vi "create data folder.vi"(7 "Book name":string="book526", 8 "error in":errorcluster, 11 "Contour plot folder":path=path "C:/Users/gyue/Box/Guang Yue uiuc research box folder/data/Contour plot") -> (0 "error out":errorcluster, 3 "xml path":path, 4 "book par":path, 5 "IV path":path, 6 "Field path":path)   [LabVIEW 2024]
panel:
  in  "Sample name":string
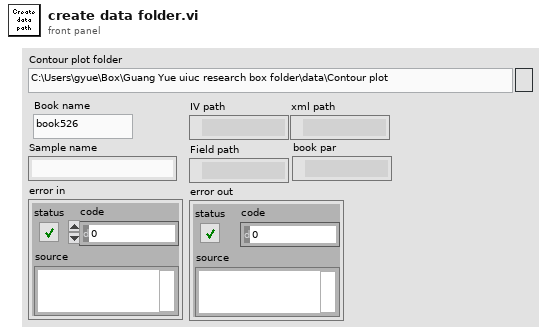
[diagram p1: front panel]
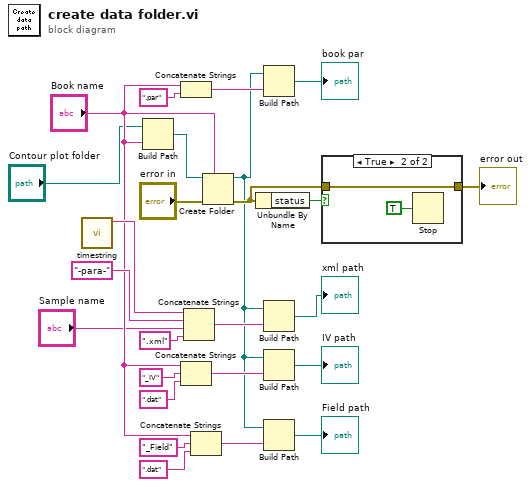
[diagram p0: block diagram]
diagram:
  n1 = call "timestring.vi"() -> ("date/time string"=w15:string)  [unwired: 11 in]
  n2 = Build Path(base path="Contour plot folder", name or relative path="Book name") -> (appended path=w18:path)
  n3 = Concatenate Strings("Book name", ".par" ("string")) -> (w20:string)
  n4 = Concatenate Strings("Book name", "_IV" ("string"), ".dat" ("string")) -> (w19:string)
  n5 = Concatenate Strings(w15, "-para-" ("string"), "Sample name", ".xml" ("string")) -> (w23:string)
  n6 = Concatenate Strings("Book name", "_Field" ("string"), ".dat" ("string")) -> (w7:string)
  n7 = Create Folder(prompt (Create Folder)="Book name", path (use dialog)=w18, error in="error in") -> (created path=w8:path, error out=w16:errorcluster)  [unwired: 1 out]
  n8 = Unbundle By Name(w16) -> ("status"=w17:bool)
  n9 = Build Path(base path=w8, name or relative path=w20) -> (appended path=→"book par":path)
  n10 = Build Path(base path=w8, name or relative path=w23) -> (appended path=→"xml path":path)
  n11 = Build Path(base path=w8, name or relative path=w19) -> (appended path=→"IV path":path)
  n12 = Build Path(base path=w8, name or relative path=w7) -> (appended path=→"Field path":path)
  n13 = case shown="True" w17 {
    tunnel: [w26 w28] -> w2
    tunnel: w16 -> [w26 w28]
    frame False {
    }
    frame True {
      n14 = Stop(stop? (T)=TRUE) -> ()
    }
  }
  "error out" <- w2
